vi "create completed tour report (minimal).vi"(1 "tour number":u64, 2 "completed_tour":T1) -> (0 "completed tour (log paragraph)":string)   [LabVIEW 2020, in "main.lvlib"]
doc: "Converts the knight tour to a paragraph of text to be logged to file."
uses:
  main.lvlib
  core/core_data/completed_tour.ctl
  core/core_data/chessboard_index.ctl
  core/core_data/tour type (enum).ctl
  core/core_data/core_data.lvlib
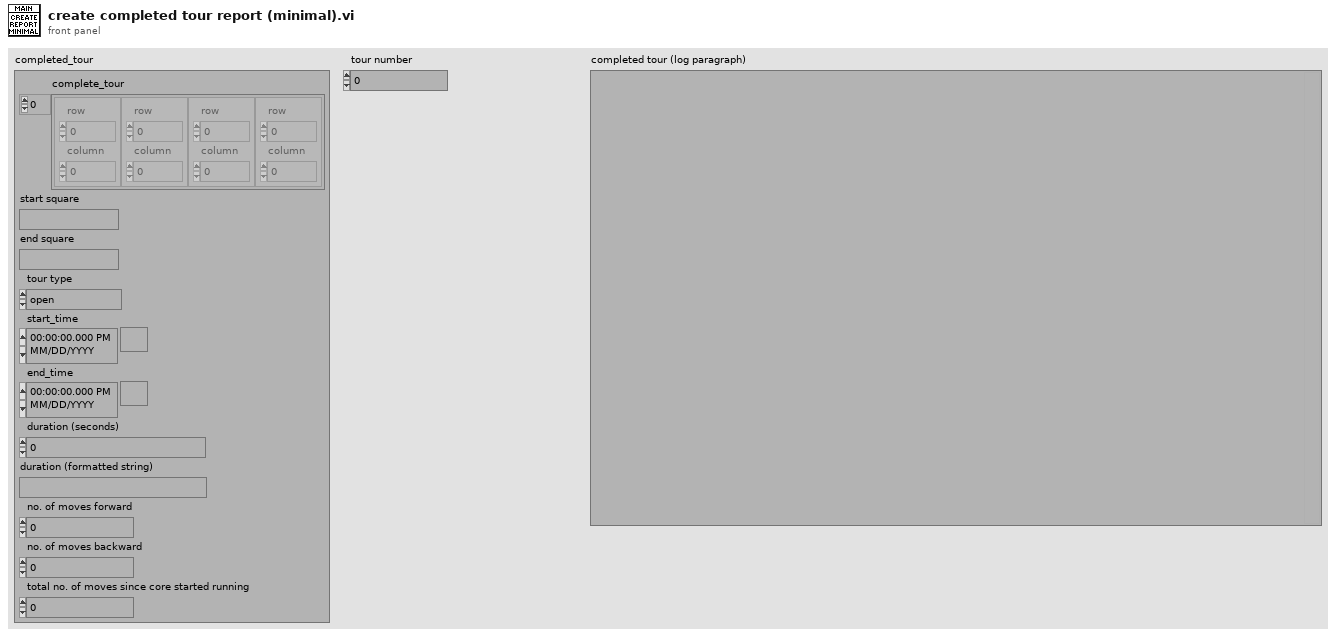
[diagram p1: front panel]
types:
  T1 = typedef "core.lvlib/core_data.lvlib/completed_tour.ctl" = cluster{"complete_tour":T2[], "start square":string, "end square":string, "tour type":T3, "start_time":timestamp, "end_time":timestamp, "duration (seconds)":dbl, "duration (formatted string)":string, "no. of moves forward":u64, "no. of moves backward":u64, "total no. of moves since core started running":u64}
  T2 = typedef "core.lvlib/core_data.lvlib/chessboard_index.ctl" = cluster{"row":u8, "column":u8}
  T3 = typedef "core.lvlib/core_data.lvlib/tour type (enum).ctl" = enum16{"open", "closed"}
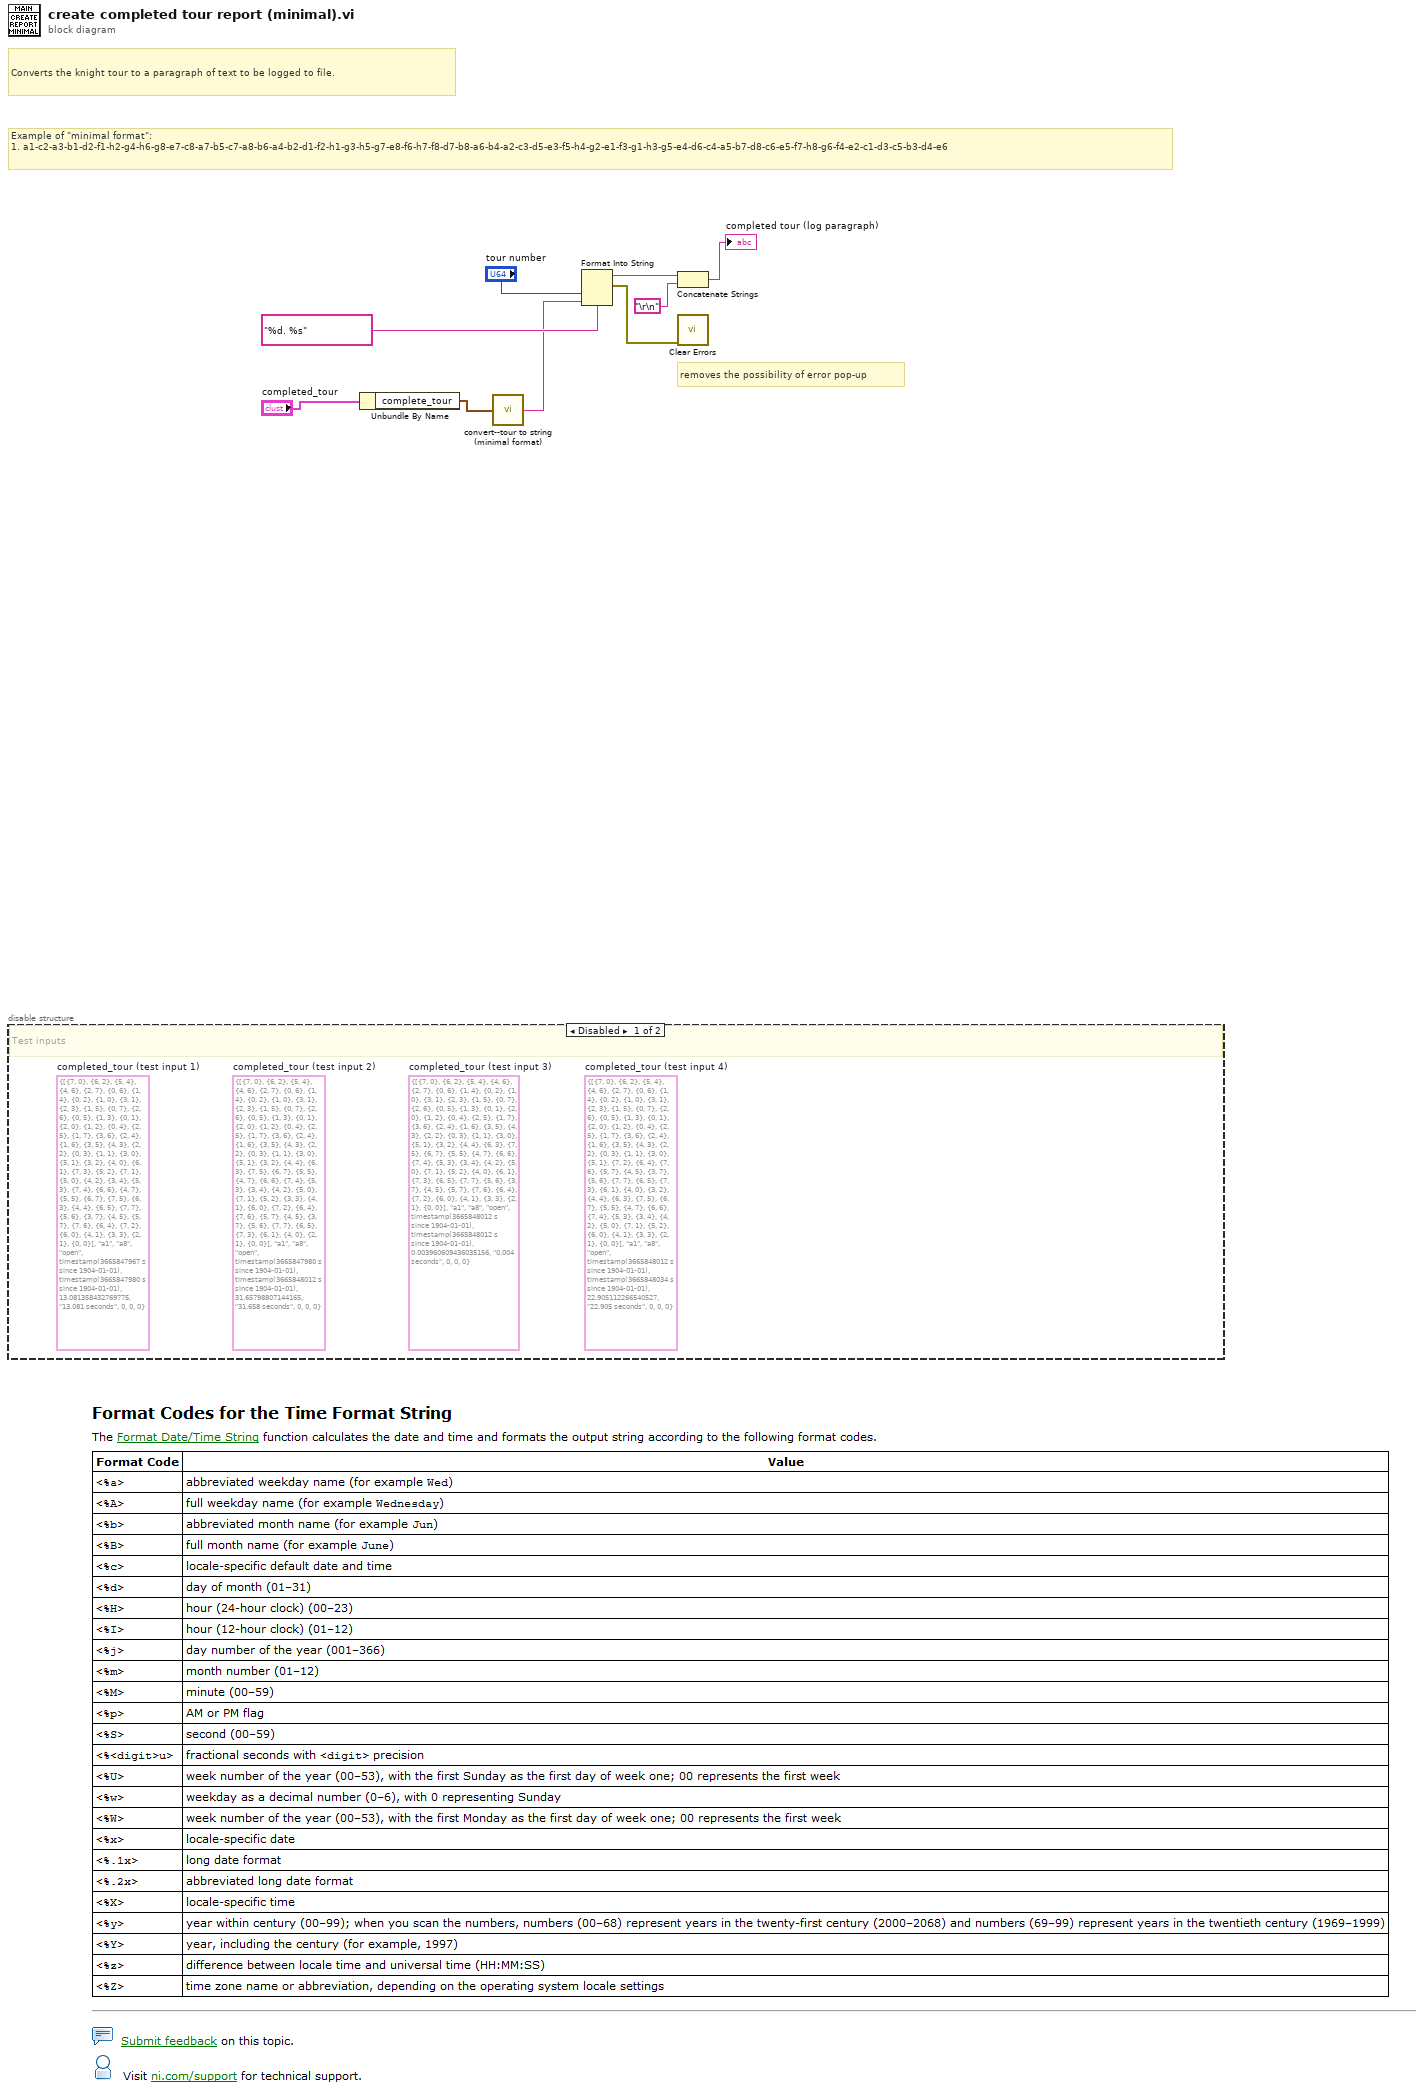
[diagram p0: block diagram]
diagram:
  # "Example of \"minimal format\":\n1. a1-c2-a3-b1-d2-f1-h2-g4-h6-g8-e7-c8-a7-b5-c7-a8-b6-a4-b2-d1-f2-h1-g3-h5-g7-e8-f6-h7-f8-d7-b8-a6-b4-a2-c3-d5-e3-f5-h4-g2-e1-f3-g1-h3-g5-e4-d6-c4-a5-b7-d8-c6-e5-f7-h8-g6-f4-e2-c1-d3-c5-b3-d4-e6"
  # "removes the possibility of error pop-up"
  # "Converts the knight tour to a paragraph of text to be logged to file."
  n1 = disable-structure shown="Disabled" {
    frame Disabled {
      (unwired) T1 {"complete_tour"=[{"row"=7, "column"=0}, {"row"=6, "column"=2}, {"row"=5, "column"=4}, {"row"=4, "column"=6}, {"row"=2, "column"=7}, {"row"=0, "column"=6}, {"row"=1, "column"=4}, {"row"=0, "column"=2}, {"row"=1, "column"=0}, {"row"=3, "column"=1}, {"row"=2, "column"=3}, {"row"=1, "column"=5}, {"row"=0, "column"=7}, {"row"=2, "column"=6}, {"row"=0, "column"=5}, {"row"=1, "column"=3}, {"row"=0, "column"=1}, {"row"=2, "column"=0}, {"row"=1, "column"=2}, {"row"=0, "column"=4}, {"row"=2, "column"=5}, {"row"=1, "column"=7}, {"row"=3, "column"=6}, {"row"=2, "column"=4}, {"row"=1, "column"=6}, {"row"=3, "column"=5}, {"row"=4, "column"=3}, {"row"=2, "column"=2}, {"row"=0, "column"=3}, {"row"=1, "column"=1}, {"row"=3, "column"=0}, {"row"=5, "column"=1}, {"row"=7, "column"=2}, {"row"=6, "column"=4}, {"row"=7, "column"=6}, {"row"=5, "column"=7}, {"row"=4, "column"=5}, {"row"=3, "column"=7}, {"row"=5, "column"=6}, {"row"=7, "column"=7}, {"row"=6, "column"=5}, {"row"=7, "column"=3}, {"row"=6, "column"=1}, {"row"=4, "column"=0}, {"row"=3, "column"=2}, {"row"=4, "column"=4}, {"row"=6, "column"=3}, {"row"=7, "column"=5}, {"row"=6, "column"=7}, {"row"=5, "column"=5}, {"row"=4, "column"=7}, {"row"=6, "column"=6}, {"row"=7, "column"=4}, {"row"=5, "column"=3}, {"row"=3, "column"=4}, {"row"=4, "column"=2}, {"row"=5, "column"=0}, {"row"=7, "column"=1}, {"row"=5, "column"=2}, {"row"=6, "column"=0}, {"row"=4, "column"=1}, {"row"=3, "column"=3}, {"row"=2, "column"=1}, {"row"=0, "column"=0}], "start square"="a1", "end square"="a8", "tour type"=enum."open", "start_time"=timestamp(3665848012.019379 s since 1904-01-01), "end_time"=timestamp(3665848034.9244914 s since 1904-01-01), "duration (seconds)"=22.905112266540527, "duration (formatted string)"="22.905 seconds", "no. of moves forward"=0, "no. of moves backward"=0, "total no. of moves since core started running"=0}  # completed_tour (test input 4)
      (unwired) T1 {"complete_tour"=[{"row"=7, "column"=0}, {"row"=6, "column"=2}, {"row"=5, "column"=4}, {"row"=4, "column"=6}, {"row"=2, "column"=7}, {"row"=0, "column"=6}, {"row"=1, "column"=4}, {"row"=0, "column"=2}, {"row"=1, "column"=0}, {"row"=3, "column"=1}, {"row"=2, "column"=3}, {"row"=1, "column"=5}, {"row"=0, "column"=7}, {"row"=2, "column"=6}, {"row"=0, "column"=5}, {"row"=1, "column"=3}, {"row"=0, "column"=1}, {"row"=2, "column"=0}, {"row"=1, "column"=2}, {"row"=0, "column"=4}, {"row"=2, "column"=5}, {"row"=1, "column"=7}, {"row"=3, "column"=6}, {"row"=2, "column"=4}, {"row"=1, "column"=6}, {"row"=3, "column"=5}, {"row"=4, "column"=3}, {"row"=2, "column"=2}, {"row"=0, "column"=3}, {"row"=1, "column"=1}, {"row"=3, "column"=0}, {"row"=5, "column"=1}, {"row"=3, "column"=2}, {"row"=4, "column"=4}, {"row"=6, "column"=3}, {"row"=7, "column"=5}, {"row"=6, "column"=7}, {"row"=5, "column"=5}, {"row"=4, "column"=7}, {"row"=6, "column"=6}, {"row"=7, "column"=4}, {"row"=5, "column"=3}, {"row"=3, "column"=4}, {"row"=4, "column"=2}, {"row"=5, "column"=0}, {"row"=7, "column"=1}, {"row"=5, "column"=2}, {"row"=4, "column"=0}, {"row"=6, "column"=1}, {"row"=7, "column"=3}, {"row"=6, "column"=5}, {"row"=7, "column"=7}, {"row"=5, "column"=6}, {"row"=3, "column"=7}, {"row"=4, "column"=5}, {"row"=5, "column"=7}, {"row"=7, "column"=6}, {"row"=6, "column"=4}, {"row"=7, "column"=2}, {"row"=6, "column"=0}, {"row"=4, "column"=1}, {"row"=3, "column"=3}, {"row"=2, "column"=1}, {"row"=0, "column"=0}], "start square"="a1", "end square"="a8", "tour type"=enum."open", "start_time"=timestamp(3665848012.0154185 s since 1904-01-01), "end_time"=timestamp(3665848012.019379 s since 1904-01-01), "duration (seconds)"=0.003960609436035156, "duration (formatted string)"="0.004 seconds", "no. of moves forward"=0, "no. of moves backward"=0, "total no. of moves since core started running"=0}  # completed_tour (test input 3)
      (unwired) T1 {"complete_tour"=[{"row"=7, "column"=0}, {"row"=6, "column"=2}, {"row"=5, "column"=4}, {"row"=4, "column"=6}, {"row"=2, "column"=7}, {"row"=0, "column"=6}, {"row"=1, "column"=4}, {"row"=0, "column"=2}, {"row"=1, "column"=0}, {"row"=3, "column"=1}, {"row"=2, "column"=3}, {"row"=1, "column"=5}, {"row"=0, "column"=7}, {"row"=2, "column"=6}, {"row"=0, "column"=5}, {"row"=1, "column"=3}, {"row"=0, "column"=1}, {"row"=2, "column"=0}, {"row"=1, "column"=2}, {"row"=0, "column"=4}, {"row"=2, "column"=5}, {"row"=1, "column"=7}, {"row"=3, "column"=6}, {"row"=2, "column"=4}, {"row"=1, "column"=6}, {"row"=3, "column"=5}, {"row"=4, "column"=3}, {"row"=2, "column"=2}, {"row"=0, "column"=3}, {"row"=1, "column"=1}, {"row"=3, "column"=0}, {"row"=5, "column"=1}, {"row"=3, "column"=2}, {"row"=4, "column"=4}, {"row"=6, "column"=3}, {"row"=7, "column"=5}, {"row"=6, "column"=7}, {"row"=5, "column"=5}, {"row"=4, "column"=7}, {"row"=6, "column"=6}, {"row"=7, "column"=4}, {"row"=5, "column"=3}, {"row"=3, "column"=4}, {"row"=4, "column"=2}, {"row"=5, "column"=0}, {"row"=7, "column"=1}, {"row"=5, "column"=2}, {"row"=3, "column"=3}, {"row"=4, "column"=1}, {"row"=6, "column"=0}, {"row"=7, "column"=2}, {"row"=6, "column"=4}, {"row"=7, "column"=6}, {"row"=5, "column"=7}, {"row"=4, "column"=5}, {"row"=3, "column"=7}, {"row"=5, "column"=6}, {"row"=7, "column"=7}, {"row"=6, "column"=5}, {"row"=7, "column"=3}, {"row"=6, "column"=1}, {"row"=4, "column"=0}, {"row"=2, "column"=1}, {"row"=0, "column"=0}], "start square"="a1", "end square"="a8", "tour type"=enum."open", "start_time"=timestamp(3665847980.3574305 s since 1904-01-01), "end_time"=timestamp(3665848012.0154185 s since 1904-01-01), "duration (seconds)"=31.65798807144165, "duration (formatted string)"="31.658 seconds", "no. of moves forward"=0, "no. of moves backward"=0, "total no. of moves since core started running"=0}  # completed_tour (test input 2)
      (unwired) T1 {"complete_tour"=[{"row"=7, "column"=0}, {"row"=6, "column"=2}, {"row"=5, "column"=4}, {"row"=4, "column"=6}, {"row"=2, "column"=7}, {"row"=0, "column"=6}, {"row"=1, "column"=4}, {"row"=0, "column"=2}, {"row"=1, "column"=0}, {"row"=3, "column"=1}, {"row"=2, "column"=3}, {"row"=1, "column"=5}, {"row"=0, "column"=7}, {"row"=2, "column"=6}, {"row"=0, "column"=5}, {"row"=1, "column"=3}, {"row"=0, "column"=1}, {"row"=2, "column"=0}, {"row"=1, "column"=2}, {"row"=0, "column"=4}, {"row"=2, "column"=5}, {"row"=1, "column"=7}, {"row"=3, "column"=6}, {"row"=2, "column"=4}, {"row"=1, "column"=6}, {"row"=3, "column"=5}, {"row"=4, "column"=3}, {"row"=2, "column"=2}, {"row"=0, "column"=3}, {"row"=1, "column"=1}, {"row"=3, "column"=0}, {"row"=5, "column"=1}, {"row"=3, "column"=2}, {"row"=4, "column"=0}, {"row"=6, "column"=1}, {"row"=7, "column"=3}, {"row"=5, "column"=2}, {"row"=7, "column"=1}, {"row"=5, "column"=0}, {"row"=4, "column"=2}, {"row"=3, "column"=4}, {"row"=5, "column"=3}, {"row"=7, "column"=4}, {"row"=6, "column"=6}, {"row"=4, "column"=7}, {"row"=5, "column"=5}, {"row"=6, "column"=7}, {"row"=7, "column"=5}, {"row"=6, "column"=3}, {"row"=4, "column"=4}, {"row"=6, "column"=5}, {"row"=7, "column"=7}, {"row"=5, "column"=6}, {"row"=3, "column"=7}, {"row"=4, "column"=5}, {"row"=5, "column"=7}, {"row"=7, "column"=6}, {"row"=6, "column"=4}, {"row"=7, "column"=2}, {"row"=6, "column"=0}, {"row"=4, "column"=1}, {"row"=3, "column"=3}, {"row"=2, "column"=1}, {"row"=0, "column"=0}], "start square"="a1", "end square"="a8", "tour type"=enum."open", "start_time"=timestamp(3665847967.276072 s since 1904-01-01), "end_time"=timestamp(3665847980.3574305 s since 1904-01-01), "duration (seconds)"=13.081358432769775, "duration (formatted string)"="13.081 seconds", "no. of moves forward"=0, "no. of moves backward"=0, "total no. of moves since core started running"=0}  # completed_tour (test input 1)
      # "Test inputs"
    }
    frame Enabled {
    }
  }
  n2 = Unbundle By Name("completed_tour") -> ("complete_tour"=w4:T2[])
  n3 = call "convert--tour to string (minimal format).vi"("tour"=w4) -> ("tour (minimal format)"=w1:string)
  n4 = Format Into String(format string="%d. %s", "tour number", w1) -> (resulting string=w8:string, error out=w6:errorcluster)  [unwired: 2 in]
  n5 = Concatenate Strings(w8, "\r\n") -> (→"completed tour (log paragraph)":string)
  n6 = call <vilib>:"Clear Errors.vi"("error in (no error)"=w6) -> ()  [unwired: 5 in, 2 out]
